vi "EPR DAQ.vi"() -> ()   [LabVIEW 2011]
uses:
  <instrlib>/niScope/Controls/niScope vertical coupling.ctl
panel:
  in  "stop":bool
  in  "?":T1(tab)
  out "Video bandwidth (Hz)":dbl
  in  "DAQ Card":refnum<k15>="PXI1Slot2"
  in  "Number of samples":i32=2000 format="%.0p"
  in  "Minimum sample rate (S/s)":dbl=100000000.0 format="%#_6p"
  in  "Reference position":dbl(slide)=50.0 scale=0.0..100.0
  in  "max time (s)":dbl=10.0 caption="Time to run (s)"
  in  "Channel parameters":T3(array[cluster])=[{"Channel name"="0", "Input impedance (Ohms)"=0, "Maximum input frequency (Hz)"=30000000.0, "vertical coupling"=1, "Probe attenuation"=1.0, "Vertical range (V)"=2.0, "Vertical offset"=0.0, "channel enabled"=TRUE}, {"Channel name"="1", "Input impedance (Ohms)"=0, "Maximum input frequency (Hz)"=30000000.0, "vertical coupling"=1, "Probe attenuation"=1.0, "Vertical range (V)"=2.0, "Vertical offset"=0.0, "channel enabled"=TRUE}] {"Input impedance (Ohms)" items=["1 mega ohm"=0, "50 ohms"=2]; "Maximum input frequency (Hz)" format="%#_6p"; "vertical coupling" items=["AC", "DC", "Ground"]}
  out "Variance 1 normalised to SNL":dbl(graph)
  out "Conditional variance":dbl(graph)
  in  "Shot noise start":bool
  out "Variance 2 normalised to SNL":dbl(graph)
  in  "Shot noise stop":bool
  in  "Record Data":bool
  in  "File location":path
  in  "Type of measurement":u16
  out "Parameters values file":string
  in  "File root name":string
  out "signal":dynamicdata(graph) caption="Signal"
  out "MS values":dbl[](graph)
  out "Actual samples acquired in waveform, ch 0":i32
  out "Loop count":i32
  out "error out":errorcluster
  out "Actual samples acquired in waveform, ch 1":i32
  # "set to -1 to fetch all available samples"
  # "Variance won't be displayed until shot noise is taken"
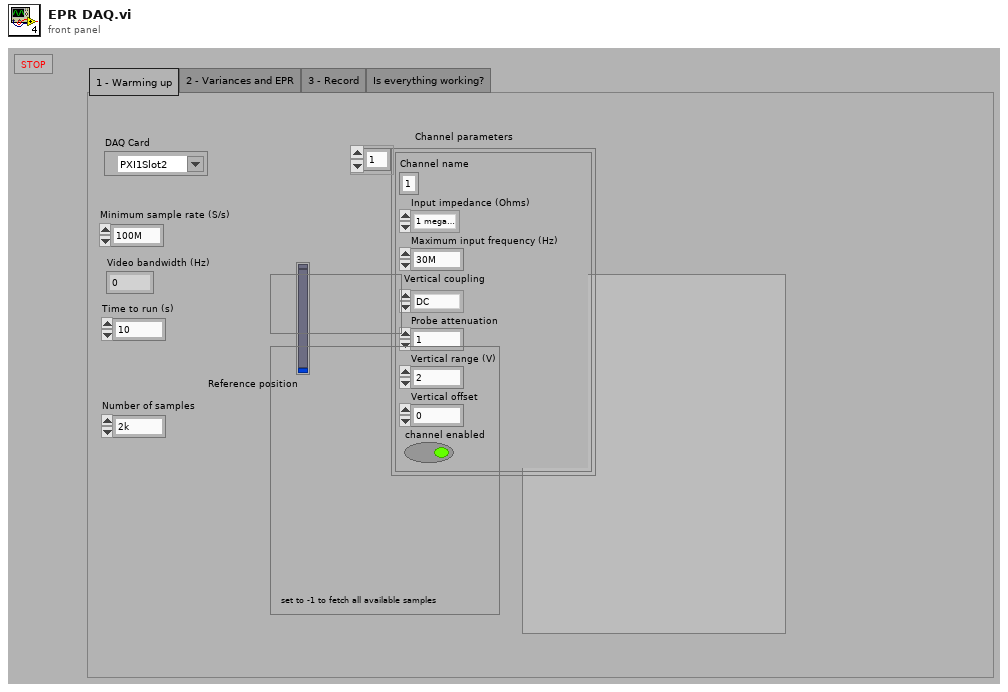
[diagram p1: front panel]
types:
  T1 = enum32{"1 - Warming up", "2 - Variances and EPR", "3 - Record", "Is everything working?"}
  T2 = typedef "niScope vertical coupling.ctl" = i32
  T3 = cluster{"Channel name":string, "Input impedance (Ohms)":u32, "Maximum input frequency (Hz)":dbl, "vertical coupling":T2, "Probe attenuation":dbl, "Vertical range (V)":dbl, "Vertical offset":dbl, "channel enabled":bool}[]
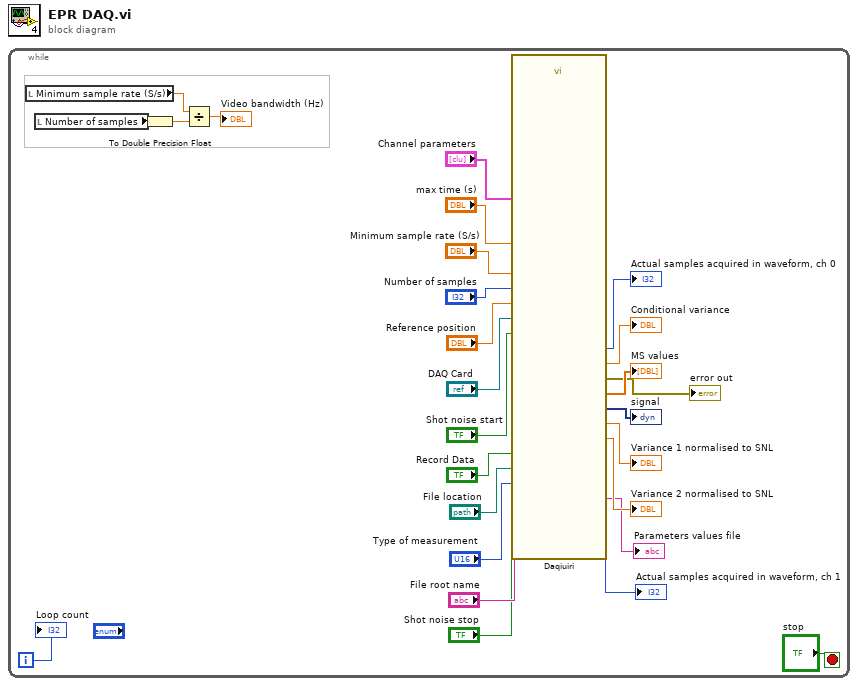
[diagram p0: block diagram]
diagram:
  n1 = while {
    i -> [w1]
    stop <- "stop" stop-if-true
    n2 = local read "Minimum sample rate (S/s)"() -> (w25:dbl)
    n3 = local read "Number of samples"() -> (w27:i32)
    n4 = To Double Precision Float(number=w27) -> (double precision float=w24:dbl)
    n5 = Divide(x=w25, y=w24) -> (x/y=→"Video bandwidth (Hz)":dbl)
    n6 = call "Daqiuiri.vi"("resource name"="DAQ Card", "Record Data"="Record Data", "numSamples"="Number of samples", "max time (s)"="max time (s)", "min sample rate"="Minimum sample rate (S/s)", "File location"="File location", "reference position"="Reference position", "Type of\nmeasurement"="Type of measurement", "Name root"="File root name", "channel parameters"="Channel parameters", "Shot noise start"="Shot noise start", "Shot noise stop"="Shot noise stop") -> ("MS values"=→"MS values":dbl[], "Variance 2 normalised to SNL"=→"Variance 2 normalised to SNL":dbl, "signal"=→"signal":dynamicdata, "Parameters values file"=→"Parameters values file":string, "Variance 1 normalised to SNL"=→"Variance 1 normalised to SNL":dbl, "actualSamples 0"=→"Actual samples acquired in waveform, ch 0":i32, "Conditional variance"=→"Conditional variance":dbl, "actualSamples 1"=→"Actual samples acquired in waveform, ch 1":i32, "error out"=→"error out":errorcluster)  [unwired: 3 in, 4 out]
    "Loop count" <- w1
  }
